vi "To-simple-string.vi"(8 "error in (no error)":errorcluster, 11 "Move-Relative in":refnum<class "Move-Relative.lvclass">) -> (0 "error out":errorcluster, 2 "Status string":string, 3 "Move-Relative out":refnum<class "Move-Relative.lvclass">)   [LabVIEW 2013, in "PowderDeposition.lvlib" / "Move-Relative.lvclass"]
uses:
  Move-Relative.lvclass
  Move-Relative.lvclass/Move-Relative.ctl
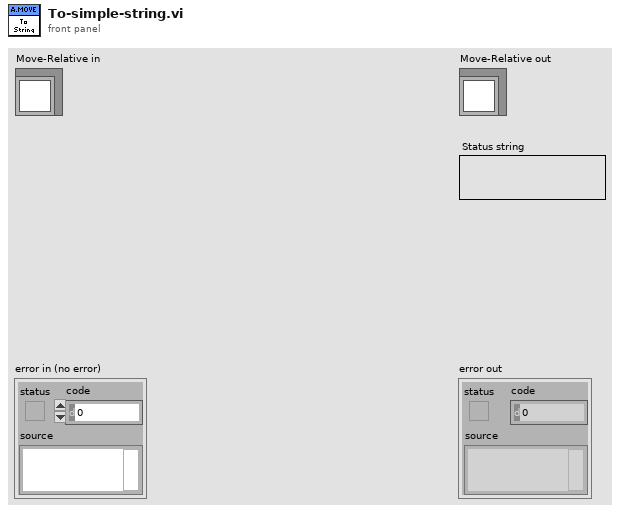
[diagram p1: front panel]
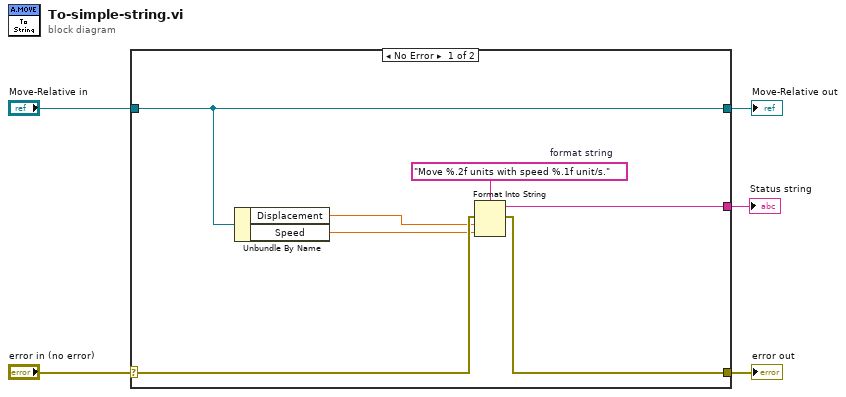
[diagram p0: block diagram]
diagram:
  n1 = case shown="No Error" "error in (no error)" {
    selector: "error in (no error)" -> [w10 w14]
    tunnel: [w11 w14] -> w4
    tunnel: [w9 w13] -> w2
    tunnel: "Move-Relative in" -> [w9 w13]
    tunnel: [w6 _] -> w1
    frame No Error {
      w12 = "Move %.2f units with speed %.1f unit/s."  # format string
      n2 = Unbundle By Name(w9) -> ("Displacement"=w7:dbl, "Speed"=w8:dbl)
      n3 = Format Into String(format string=w12, error in=w10, w7, w8) -> (resulting string=w6:string, error out=w11:errorcluster)  [unwired: 1 in]
    }
    frame Error {
    }
  }
  "error out" <- w4
  "Move-Relative out" <- w2
  "Status string" <- w1
